vi "Run Bfr Rx - Cached - Add to Cache.vi"(5 "Data Offset in":u64, 7 "Data in":u8[](array[numeric]), 8 "error in (no error)":errorcluster, 11 "Cache Buffer":u64 format="%016x") -> (0 "error out":errorcluster)   [LabVIEW 2021, in "UDP-Custom-Device Engine.lvlib"]
uses:
  UDP-Custom-Device Engine.lvlib
  <vilib>/NI VeriStand/VeriStand Data/Pointer Operations/Pointer.Write (1D U8).vi
  <vilib>/NI VeriStand/VeriStand Data/VeriStand Data.lvlib
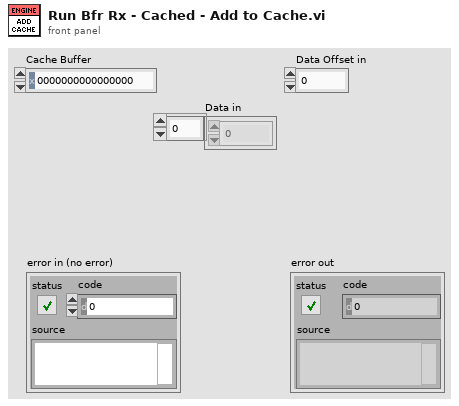
[diagram p1: front panel]
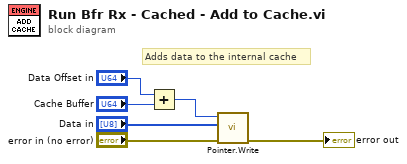
[diagram p0: block diagram]
diagram:
  # "Adds data to the internal cache"
  n1 = Add(x="Data Offset in", y="Cache Buffer") -> (x+y=w2:u64)
  n2 = call-poly <vilib>:"Pointer.Write.vi"("error in (no error)"="error in (no error)", "values"="Data in", "pointer in"=w2) -> ("error out"=→"error out":errorcluster)  [unwired: 6 in, 2 out]
